vi "Write Variant Data.vi"(8 "error in (no error)":errorcluster, 10 "data":variant, 11 "My Custom Type in":refnum<class "My Custom Type.lvclass">) -> (0 "error out":errorcluster, 3 "My Custom Type out":refnum<class "My Custom Type.lvclass">)   [LabVIEW 2020, in "My Custom Type.lvclass"]
uses:
  My Custom Type.lvclass
  My Custom Type.lvclass/My Custom Type.ctl
  source/PV Data/EPICS Time Stamp.ctl
  source/PV Data/PV Data.lvlib
  Custom Structure.ctl
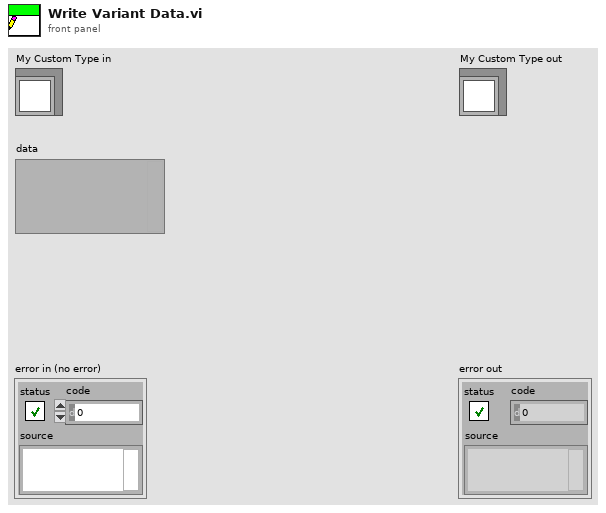
[diagram p1: front panel]
types:
  T1 = typedef "Custom Structure.ctl" = cluster{"fieldA":i32, "fieldB":string, "fieldC":cluster{"fieldC1":bool, "fieldC2":dbl}, "timeStamp":T2}
  T2 = typedef "PV Access.lvlib/PV Data.lvlib/EPICS Time Stamp.ctl" = cluster{"secondsPastEpoch":i64, "nanoseconds":i32, "userTag":i32}
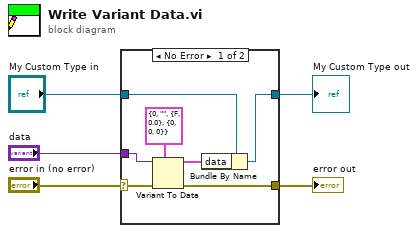
[diagram p0: block diagram]
diagram:
  n1 = case shown="No Error" "error in (no error)" {
    selector: "error in (no error)" -> [w8 w13]
    tunnel: "My Custom Type in" -> [w12 w14]
    tunnel: "data" -> [w9 _]
    tunnel: [w7 w13] -> w2
    tunnel: [w6 w14] -> w1
    frame No Error {
      n2 = Variant To Data(error in=w8, type=T1 {"fieldA"=0, "fieldB"="", "fieldC"={"fieldC1"=FALSE, "fieldC2"=0.0}, "timeStamp"={"secondsPastEpoch"=0, "nanoseconds"=0, "userTag"=0}} ("Cluster"), Variant=w9) -> (data=w10:T1, error out=w7:errorcluster)
      n3 = Bundle By Name(cluster=w12, "data"=w10) -> (w6:refnum<class "My Custom Type.lvclass">)
    }
    frame Error {
    }
  }
  "error out" <- w2
  "My Custom Type out" <- w1
